vi "Next Capture.vi"   [LabVIEW 2020, in "capture.lvlib" / "Stream.lvclass"]
uses:
  Stream.lvclass
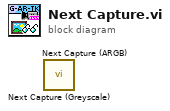
[diagram p0: block diagram]
diagram:
  n1 = call "Next Capture (Greyscale).vi"() -> ()  [unwired: 8 in, 4 out]
  n2 = call "Next Capture (ARGB).vi"() -> ()  [unwired: 8 in, 4 out]
